vi "Timing Facade.vi"(0 "Data In":T4, 2 "Display State In":T2, 3 "Container State":T3) -> (6 "Data Out":T4, 7 "Display State Out":T2, 8 "Action":T1)   [LabVIEW 2012, in "Time Slider.xctl"]
uses:
  Time Slider.xctl
  Timing Data.ctl
  <vilib>/_xctls/Container State.ctl
  Timing State.ctl
  <vilib>/_xctls/Action.ctl
  <vilib>/_xctls/XControlSupport.lvlib
panel:
  in  "Off-Time":bool
  in  "On-Time":bool
  in  "SEQ 1":cluster{dbl, dbl, dbl}(slide) scale=0.0..20.0 scale format="%#.2f"
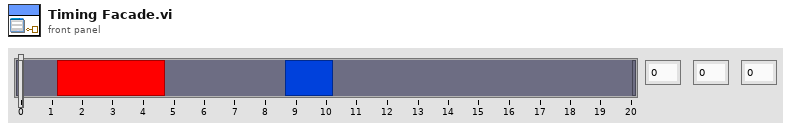
[diagram p1: front panel]
types:
  T1 = typedef "XControlSupport.lvlib/Action.ctl" = cluster{"Data Changed?":bool, "State Changed?":bool, "Action Name":string}
  T2 = typedef "Time Slider.xctl/Timing State.ctl" = cluster{"Range Max":dbl, "Range Min":dbl}
  T3 = typedef "XControlSupport.lvlib/Container State.ctl" = cluster{"Indicator?":bool, "Run Mode?":bool, " Refnum":refnum<vi>}
  T4 = typedef "Time Slider.xctl/Timing Data.ctl" = cluster{"Data":dbl, "Data 2":dbl, "Data 3":dbl}
  T5 = cluster{"Old Slider Values":dbl[], "Mouse Down Left":i32, "Old Controls Left":i32[], "Drag?":bool}
  T6 = enum8{"Enabled", "Disabled", "Disabled and Grayed Out"}
  T7 = typedef "LVPoint32TypeDef.ctl" = cluster{"Horizontal":i32, "Vertical":i32}
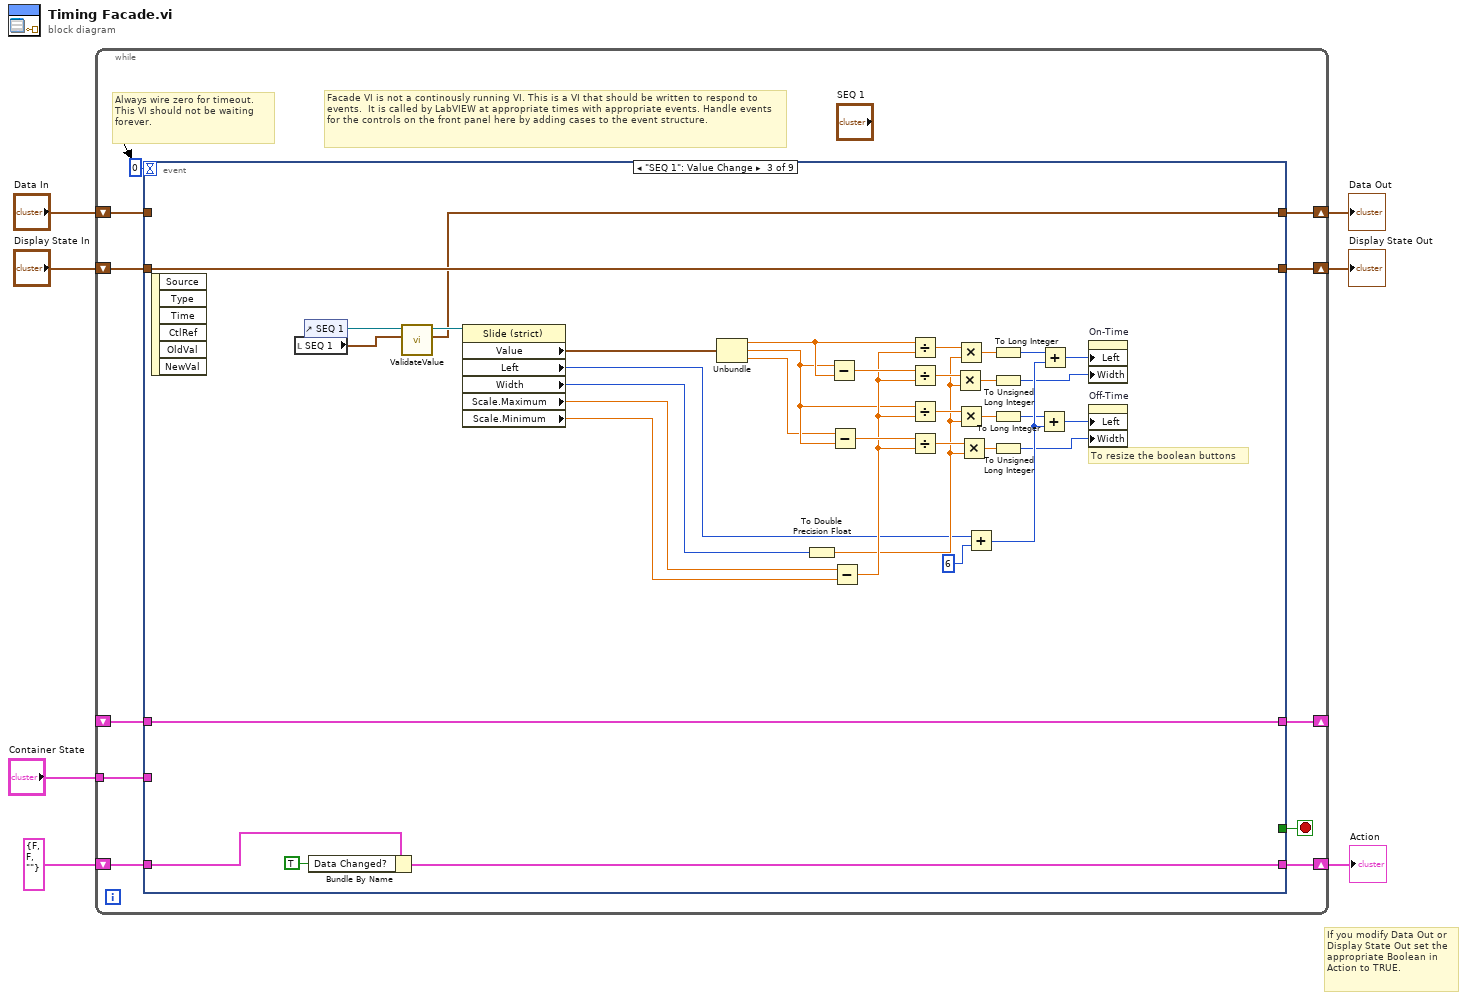
[diagram p0: block diagram]
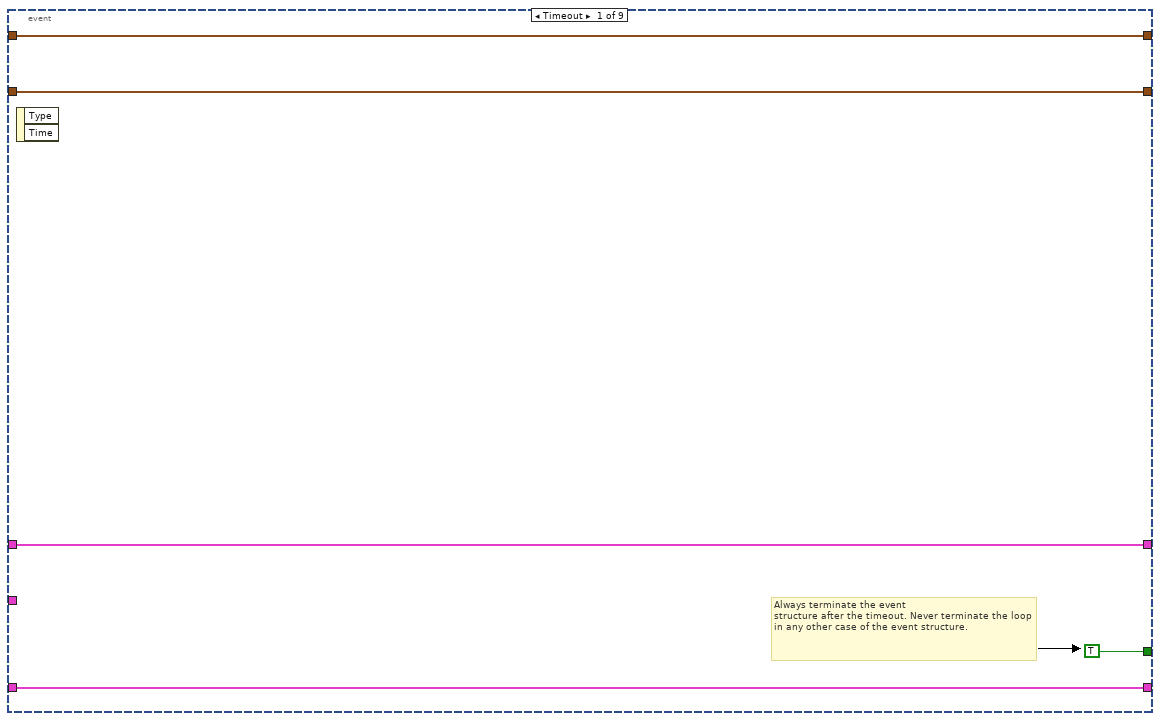
[diagram p2: hidden frame]
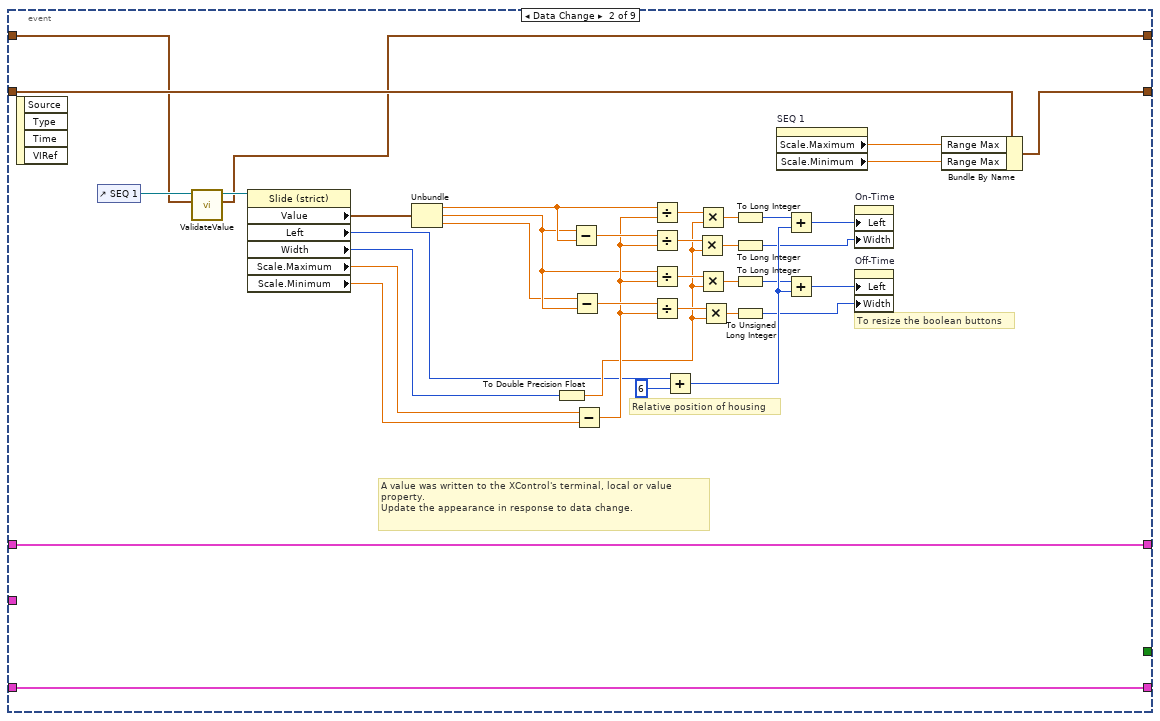
[diagram p3: hidden frame]
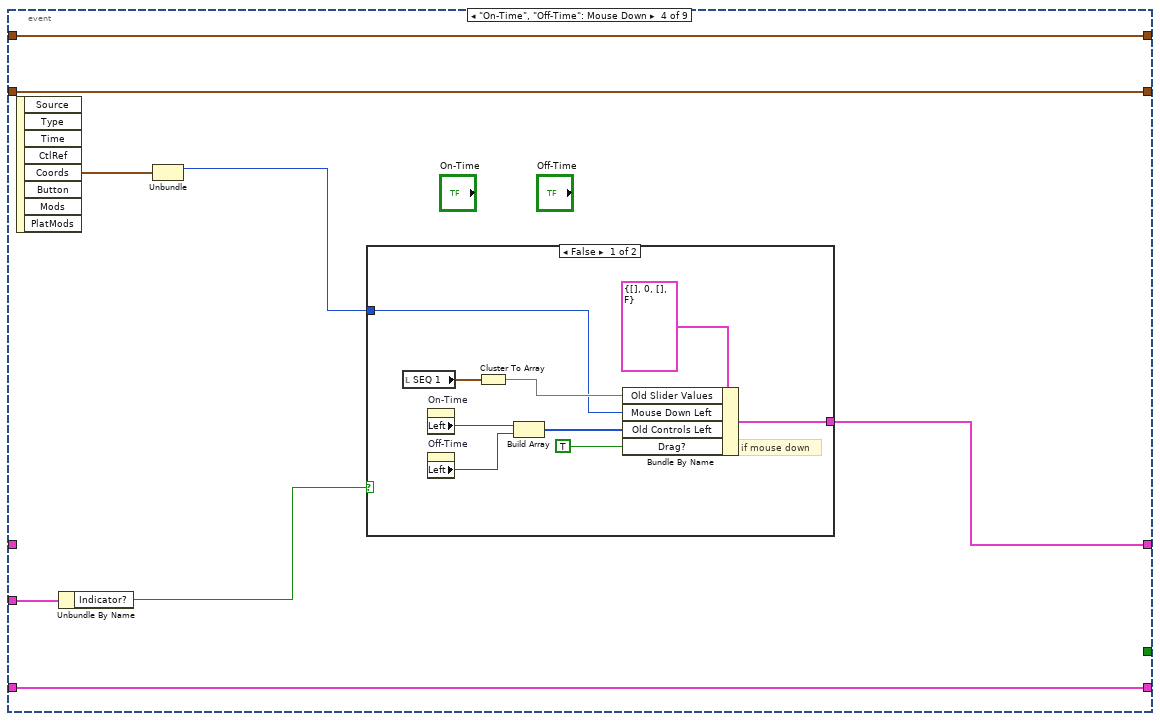
[diagram p4: hidden frame]
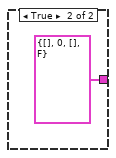
[diagram p5: hidden frame]
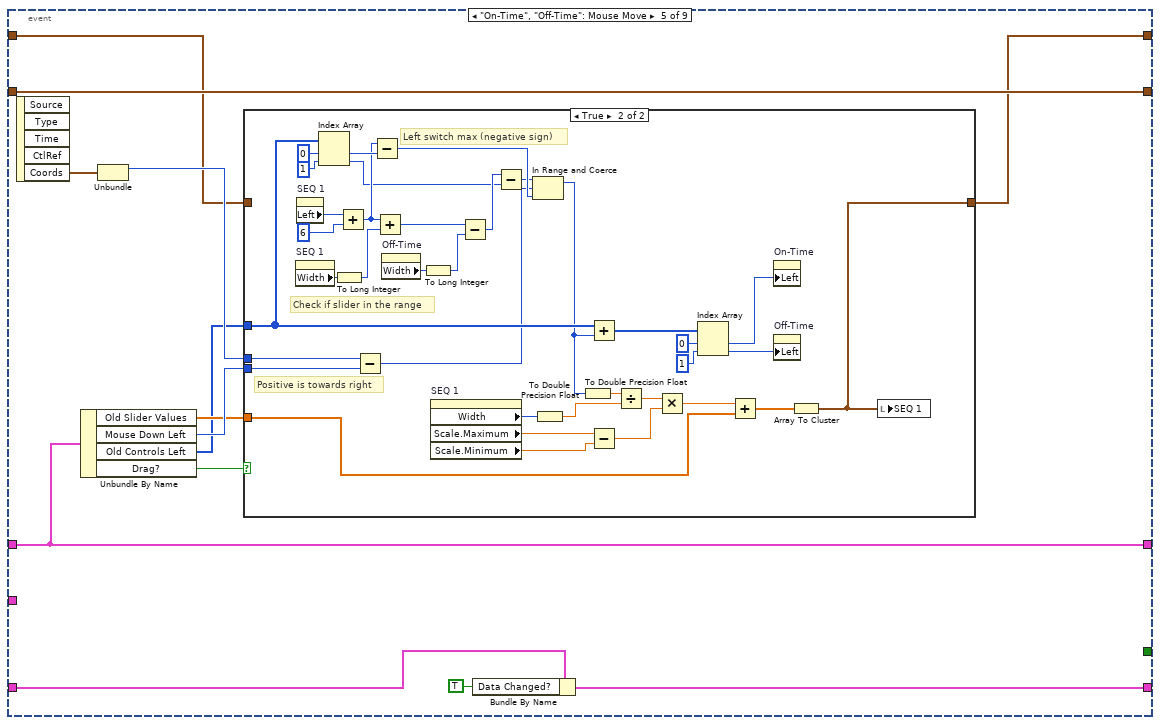
[diagram p6: hidden frame]
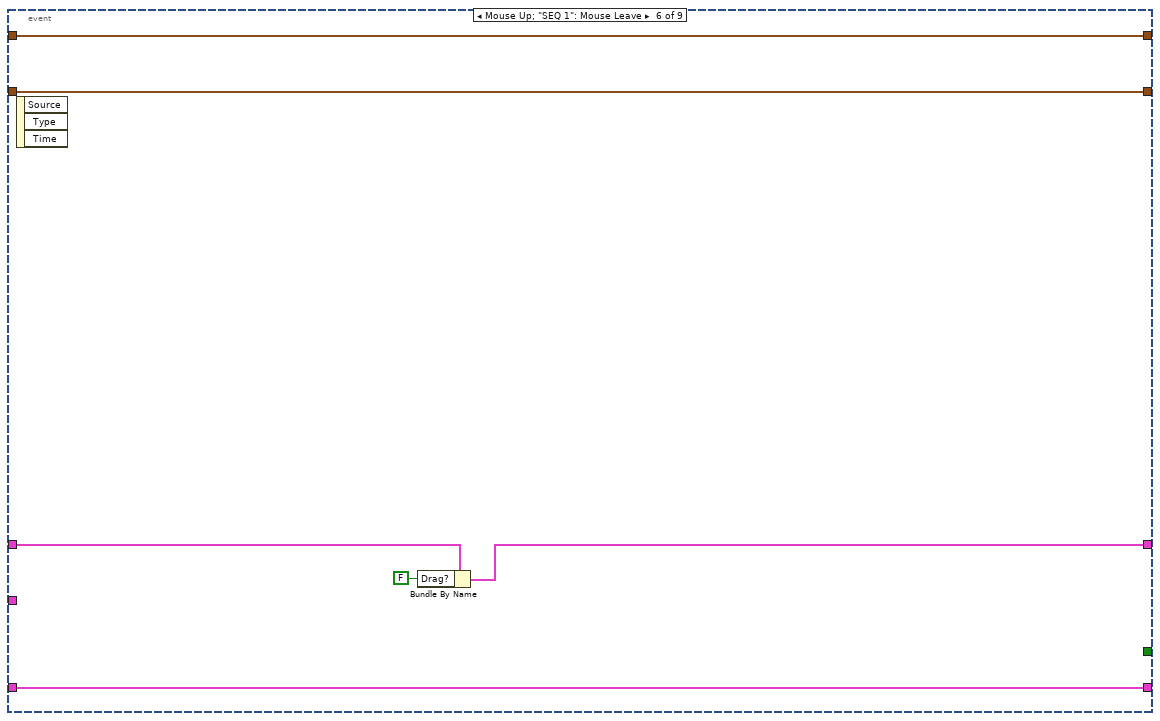
[diagram p8: hidden frame]
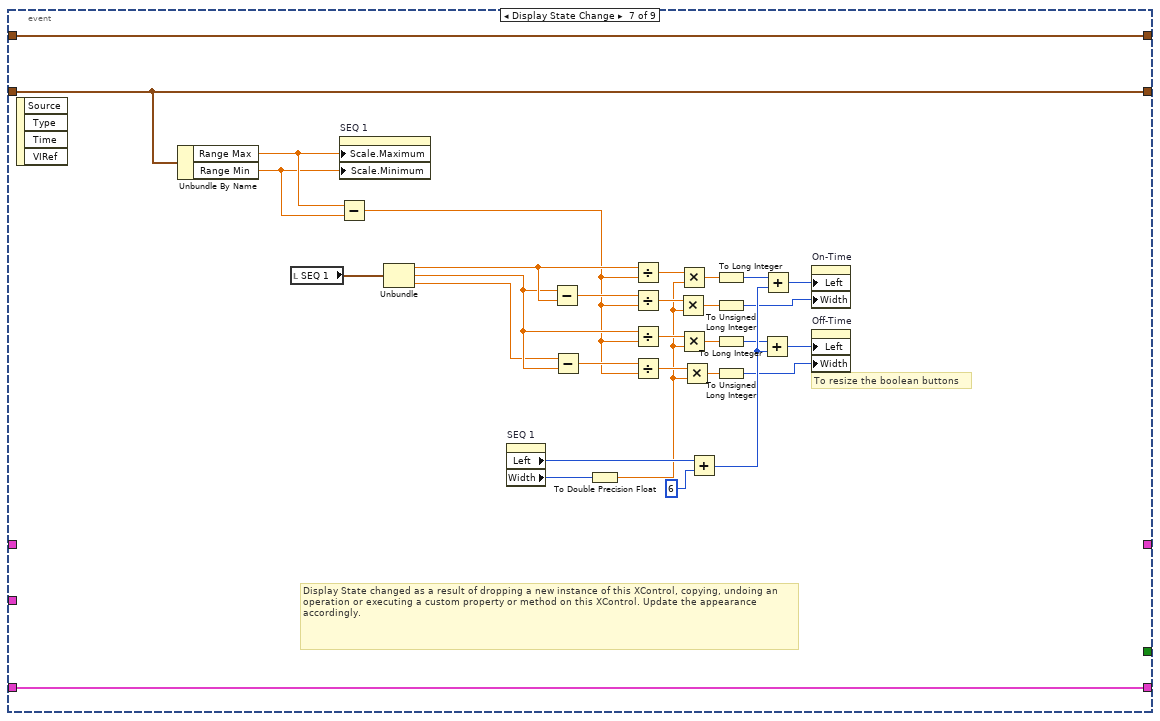
[diagram p9: hidden frame]
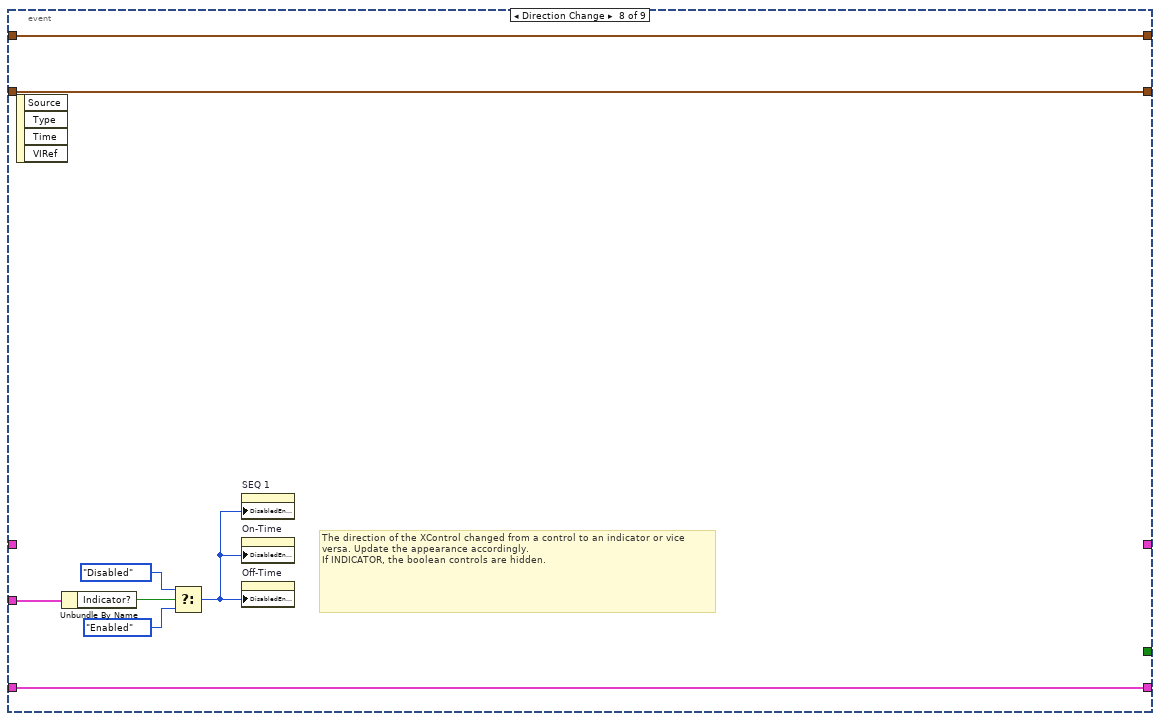
[diagram p10: hidden frame]
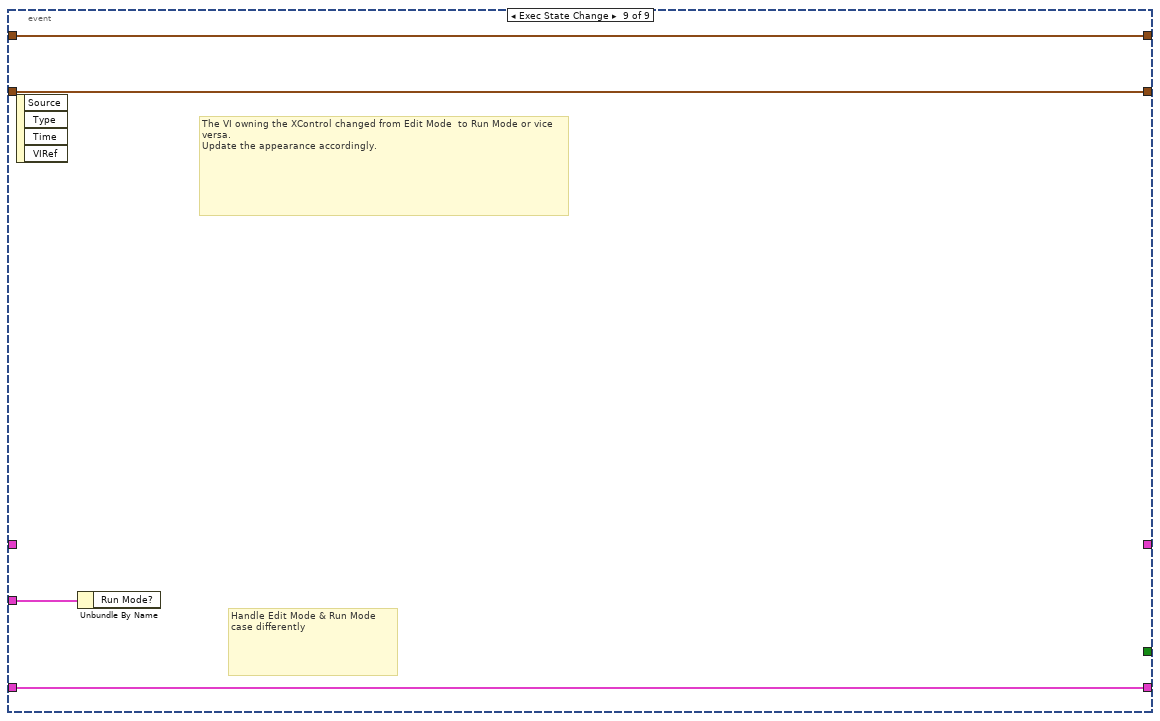
[diagram p11: hidden frame]
diagram:
  # "If you modify Data Out or Display State Out set the appropriate Boolean in Action to TRUE."
  n1 = while {
    shift-right: [w17] -> w4
    shift-left: "Display State In" -> [w18]
    tunnel: "Container State" -> [w14]
    shift-right: [w12] -> w7
    shift-left: "Data In" -> [w13]
    shift-right: [w10] -> w2
    shift-left: T1 {"Data Changed?"=FALSE, "State Changed?"=FALSE, "Action Name"=""} ("Action") -> [w11]
    shift-right: [w9] -> _
    shift-left: _ -> [w8]
    stop <- w16 stop-if-true
    # "Facade VI is not a continously running VI. This is a VI that should be written to respond to events.  It is called by LabVIEW at appropriate times with appropriate events. Handle events for the controls on the front panel here by adding cases to the event structure."
    # "Always wire zero for timeout. This VI should not be waiting forever."
    n2 = event shown="[2] \"SEQ 1\": Value Change" {
      selector: _ -> [_ _ _ _ _ _ _ _ _]
      dyn-events: _ -> [_ _ _ _ _ _ _ _ _]
      timeout: 0 -> [_ _ _ _ _ _ _ _ _]
      tunnel: w18 -> [w19 w37 w98 w106 w129 w172 w201 w210 w214]
      tunnel: [w19 w36 w98 w106 w129 w172 w201 w210 w214] -> w17
      tunnel: [TRUE _ _ _ _ _ _ _ _] -> w16
      tunnel: w14 -> [_ _ _ w103 _ _ _ w211 w215]
      tunnel: w13 -> [w21 w33 _ w104 w124 w171 w203 w209 w213]
      tunnel: [w21 w25 w63 w104 w123 w171 w203 w209 w213] -> w12
      tunnel: [w22 w61 w82 w99 w117 w167 w202 w208 w212] -> w10
      tunnel: w11 -> [w22 w61 w83 w99 w118 w167 w202 w208 w212]
      tunnel: [w20 w46 w79 w105 w121 w168 _ _ _] -> w9
      tunnel: w8 -> [w20 w46 w79 _ w121 w170 _ _ _]
      event Timeout {
        # "Always terminate the event\nstructure after the timeout. Never terminate the loop in any other case of the event structure."
        n3 = event-data() -> ()  [unwired: 1 in, 2 out]
      }
      event Data Change {
        # "Relative position of housing"
        # "To resize the boolean buttons"
        # "A value was written to the XControl's terminal, local or value property.\nUpdate the appearance in response to data change."
        n4 = event-data() -> ()  [unwired: 1 in, 4 out]
        n5 = control-ref of="SEQ 1"() -> (w34:refnum<vi>)
        n6 = call "ValidateValue.vi"("SEQ 1"=w33, "Slide Refnum in"=w34) -> ("SEQ out"=w25:cluster{dbl, dbl, dbl}, "Slide Refnum out"=w35:refnum<vi>)  [unwired: 8 in]
        n7 = property class="Slide (strict)"(reference=w35) -> ("Value"=w24:cluster{dbl, dbl, dbl}, "Left"=w29:i32, "Width"=w28:u32, "Scale.Maximum"=w27:dbl, "Scale.Minimum"=w26:dbl)  [unwired: 1 in, 2 out]
        n8 = Unbundle(w24) -> (w32:dbl, w31:dbl, w30:dbl)
        n9 = To Double Precision Float(number=w28) -> (double precision float=w45:dbl)
        n10 = Subtract(x=w31, y=w32) -> (x-y=w60:dbl)
        n11 = Subtract(x=w30, y=w31) -> (x-y=w57:dbl)
        n12 = Subtract(x=w27, y=w26) -> (x-y=w48:dbl)
        n13 = Divide(x=w32, y=w48) -> (x/y=w54:dbl)
        n14 = Divide(x=w60, y=w48) -> (x/y=w59:dbl)
        n15 = Divide(x=w31, y=w48) -> (x/y=w51:dbl)
        n16 = Divide(x=w57, y=w48) -> (x/y=w56:dbl)
        n17 = Add(x=w29, y=6) -> (x+y=w47:i32)
        n18 = Multiply(x=w59, y=w45) -> (x*y=w58:dbl)
        n19 = Multiply(x=w54, y=w45) -> (x*y=w53:dbl)
        n20 = Multiply(x=w51, y=w45) -> (x*y=w50:dbl)
        n21 = Multiply(x=w56, y=w45) -> (x*y=w55:dbl)
        n22 = To Long Integer(number=w53) -> (32bit integer=w44:i32)
        n23 = To Long Integer(number=w58) -> (32bit integer=w40:i32)
        n24 = To Long Integer(number=w50) -> (32bit integer=w42:i32)
        n25 = To Unsigned Long Integer(number=w55) -> (unsigned 32bit integer=w41:u32)
        n26 = property on="SEQ 1" class="Slide (strict)"() -> ("Scale.Maximum"=w39:dbl, "Scale.Minimum"=w38:dbl)  [unwired: 2 in, 2 out]
        n27 = Add(x=w44, y=w47) -> (x+y=w52:i32)
        n28 = Add(x=w42, y=w47) -> (x+y=w49:i32)
        n29 = property on="On-Time" class="Bool (strict)"("Left"=w52, "Width"=w40) -> ()  [unwired: 2 in, 2 out]
        n30 = property on="Off-Time" class="Bool (strict)"("Left"=w49, "Width"=w41) -> ()  [unwired: 2 in, 2 out]
        n31 = Bundle By Name(cluster=w37, "Range Max"=w39, "Range Max"=w38) -> (w36:T2)
      }
      event "SEQ 1": Value Change {
        # "To resize the boolean buttons"
        n32 = event-data() -> ()  [unwired: 1 in, 6 out]
        n33 = local read "SEQ 1"() -> (w73:cluster{dbl, dbl, dbl})
        n34 = control-ref of="SEQ 1"() -> (w72:refnum<vi>)
        n35 = Bundle By Name(cluster=w83, "Data Changed?"=TRUE) -> (w82:T1)
        n36 = call "ValidateValue.vi"("SEQ 1"=w73, "Slide Refnum in"=w72) -> ("SEQ out"=w63:cluster{dbl, dbl, dbl}, "Slide Refnum out"=w68:refnum<vi>)  [unwired: 8 in]
        n37 = property class="Slide (strict)"(reference=w68) -> ("Value"=w62:cluster{dbl, dbl, dbl}, "Left"=w67:i32, "Width"=w66:u32, "Scale.Maximum"=w65:dbl, "Scale.Minimum"=w64:dbl)  [unwired: 1 in, 2 out]
        n38 = Unbundle(w62) -> (w71:dbl, w70:dbl, w69:dbl)
        n39 = To Double Precision Float(number=w66) -> (double precision float=w78:dbl)
        n40 = Subtract(x=w70, y=w71) -> (x-y=w97:dbl)
        n41 = Subtract(x=w69, y=w70) -> (x-y=w94:dbl)
        n42 = Subtract(x=w65, y=w64) -> (x-y=w85:dbl)
        n43 = Divide(x=w71, y=w85) -> (x/y=w91:dbl)
        n44 = Divide(x=w97, y=w85) -> (x/y=w96:dbl)
        n45 = Divide(x=w70, y=w85) -> (x/y=w88:dbl)
        n46 = Divide(x=w94, y=w85) -> (x/y=w93:dbl)
        n47 = Multiply(x=w96, y=w78) -> (x*y=w95:dbl)
        n48 = Multiply(x=w91, y=w78) -> (x*y=w90:dbl)
        n49 = Multiply(x=w88, y=w78) -> (x*y=w87:dbl)
        n50 = Multiply(x=w93, y=w78) -> (x*y=w92:dbl)
        n51 = Add(x=w67, y=6) -> (x+y=w81:i32)
        n52 = To Long Integer(number=w90) -> (32bit integer=w77:i32)
        n53 = To Unsigned Long Integer(number=w95) -> (unsigned 32bit integer=w75:u32)
        n54 = To Long Integer(number=w87) -> (32bit integer=w76:i32)
        n55 = To Unsigned Long Integer(number=w92) -> (unsigned 32bit integer=w74:u32)
        n56 = Add(x=w76, y=w81) -> (x+y=w86:i32)
        n57 = Add(x=w77, y=w81) -> (x+y=w89:i32)
        n58 = property on="On-Time" class="Bool (strict)"("Left"=w89, "Width"=w75) -> ()  [unwired: 2 in, 2 out]
        n59 = property on="Off-Time" class="Bool (strict)"("Left"=w86, "Width"=w74) -> ()  [unwired: 2 in, 2 out]
      }
      event "On-Time", "Off-Time": Mouse Down {
        n60 = event-data() -> ("Coords"=w101:T7)  [unwired: 1 in, 7 out]
        n61 = Unbundle By Name(w103) -> ("Indicator?"=w102:bool)
        n62 = Unbundle(w101) -> ("Horizontal"=w100:i32)  [unwired: 1 out]
        n63 = case shown="False" w102 {
          tunnel: [w114 T5 {"Old Slider Values"=[], "Mouse Down Left"=0, "Old Controls Left"=[], "Drag?"=FALSE}] -> w105
          tunnel: w100 -> [w107 _]
          frame False {
            # "if mouse down"
            n64 = local read "SEQ 1"() -> (w108:cluster{dbl, dbl, dbl})
            n65 = property on="On-Time" class="Bool (strict)"() -> ("Left"=w112:i32)  [unwired: 2 in, 2 out]
            n66 = property on="Off-Time" class="Bool (strict)"() -> ("Left"=w111:i32)  [unwired: 2 in, 2 out]
            n67 = Cluster To Array(cluster=w108) -> (array=w109:dbl[])
            n68 = Build Array(w112, w111) -> (w110:i32[])
            n69 = Bundle By Name(cluster=T5 {"Old Slider Values"=[], "Mouse Down Left"=0, "Old Controls Left"=[], "Drag?"=FALSE}, "Old Slider Values"=w109, "Mouse Down Left"=w107, "Old Controls Left"=w110, "Drag?"=TRUE) -> (w114:T5)
          }
          frame True {
          }
        }
      }
      event "On-Time", "Off-Time": Mouse Move {
        n70 = event-data() -> ("Coords"=w128:T7)  [unwired: 1 in, 4 out]
        n71 = Unbundle By Name(w121) -> ("Old Slider Values"=w122:dbl[], "Mouse Down Left"=w125:i32, "Old Controls Left"=w120:i32[], "Drag?"=w126:bool)
        n72 = Unbundle(w128) -> ("Horizontal"=w127:i32)  [unwired: 1 out]
        n73 = case shown="True" w126 {
          tunnel: w127 -> [_ w166]
          tunnel: w125 -> [_ w165]
          tunnel: w120 -> [_ w148]
          tunnel: w124 -> [w130 _]
          tunnel: [w130 w153] -> w123
          tunnel: w122 -> [_ w152]
          frame False {
          }
          frame True {
            # "Positive is towards right"
            # "Left switch max (negative sign)"
            # "Check if slider in the range"
            n74 = property on="SEQ 1" class="Slide (strict)"() -> ("Width"=w141:u32)  [unwired: 2 in, 2 out]
            n75 = property on="SEQ 1" class="Slide (strict)"() -> ("Left"=w151:i32)  [unwired: 2 in, 2 out]
            n76 = Index Array(array=w148, index #1=0 ("index"), index #2=1 ("index")) -> (element #1=w143:i32, element #2=w137:i32)
            n77 = To Long Integer(number=w141) -> (32bit integer=w134:i32)
            n78 = Add(x=w151, y=6) -> (x+y=w142:i32)
            n79 = Subtract(x=w166, y=w165) -> (x-y=w144:i32)
            n80 = Subtract(x=w142, y=w143) -> (x-y=w145:i32)
            n81 = Add(x=w142, y=w134) -> (x+y=w139:i32)
            n82 = property on="Off-Time" class="Bool (strict)"() -> ("Width"=w140:u32)  [unwired: 2 in, 2 out]
            n83 = To Long Integer(number=w140) -> (32bit integer=w133:i32)
            n84 = property on="SEQ 1" class="Slide (strict)"() -> ("Width"=w160:u32, "Scale.Maximum"=w156:dbl, "Scale.Minimum"=w155:dbl)  [unwired: 2 in, 2 out]
            n85 = Subtract(x=w139, y=w133) -> (x-y=w138:i32)
            n86 = Subtract(x=w138, y=w137) -> (x-y=w136:i32)
            n87 = In Range and Coerce(upper limit=w136, x=w144, lower limit=w145) -> (coerced(x)=w135:i32)  [unwired: 1 out]
            n88 = To Double Precision Float(number=w160) -> (double precision float=w132:dbl)
            n89 = To Double Precision Float(number=w135) -> (double precision float=w131:dbl)
            n90 = Add(x=w148, y=w135) -> (x+y=w164:i32[])
            n91 = Subtract(x=w156, y=w155) -> (x-y=w154:dbl)
            n92 = Divide(x=w131, y=w132) -> (x/y=w159:dbl)
            n93 = Multiply(x=w159, y=w154) -> (x*y=w158:dbl)
            n94 = Index Array(array=w164, index #1=0 ("index"), index #2=1 ("index")) -> (element #1=w149:i32, element #2=w161:i32)
            n95 = Add(x=w158, y=w152) -> (x+y=w157:dbl[])
            n96 = property on="On-Time" class="Bool (strict)"("Left"=w149) -> ()  [unwired: 2 in, 2 out]
            n97 = property on="Off-Time" class="Bool (strict)"("Left"=w161) -> ()  [unwired: 2 in, 2 out]
            n98 = Array To Cluster(array=w157) -> (cluster=w153:cluster{"[0]":dbl, "[1]":dbl, "[2]":dbl})
            n99 = local write "SEQ 1"(w153) -> ()
          }
        }
        n100 = Bundle By Name(cluster=w118, "Data Changed?"=TRUE) -> (w117:T1)
      }
      event Mouse Up; "SEQ 1": Mouse Leave {
        n101 = event-data() -> ()  [unwired: 1 in, 3 out]
        n102 = Bundle By Name(cluster=w170, "Drag?"=FALSE) -> (w168:T5)
      }
      event Display State Change {
        # "To resize the boolean buttons"
        # "Display State changed as a result of dropping a new instance of this XControl, copying, undoing an operation or executing a custom property or method on this XControl. Update the appearance accordingly."
        n103 = event-data() -> ()  [unwired: 1 in, 4 out]
        n104 = Unbundle By Name(w201) -> ("Range Max"=w175:dbl, "Range Min"=w174:dbl)
        n105 = local read "SEQ 1"() -> (w179:cluster{dbl, dbl, dbl})
        n106 = Subtract(x=w175, y=w174) -> (x-y=w173:dbl)
        n107 = property on="SEQ 1" class="Slide (strict)"("Scale.Maximum"=w175, "Scale.Minimum"=w174) -> ()  [unwired: 2 in, 2 out]
        n108 = Unbundle(w179) -> (w178:dbl, w177:dbl, w176:dbl)
        n109 = property on="SEQ 1" class="Slide (strict)"() -> ("Left"=w187:i32, "Width"=w188:u32)  [unwired: 2 in, 2 out]
        n110 = Subtract(x=w177, y=w178) -> (x-y=w200:dbl)
        n111 = Subtract(x=w176, y=w177) -> (x-y=w197:dbl)
        n112 = To Double Precision Float(number=w188) -> (double precision float=w184:dbl)
        n113 = Divide(x=w178, y=w173) -> (x/y=w194:dbl)
        n114 = Divide(x=w200, y=w173) -> (x/y=w199:dbl)
        n115 = Divide(x=w177, y=w173) -> (x/y=w191:dbl)
        n116 = Divide(x=w197, y=w173) -> (x/y=w196:dbl)
        n117 = Multiply(x=w199, y=w184) -> (x*y=w198:dbl)
        n118 = Multiply(x=w194, y=w184) -> (x*y=w193:dbl)
        n119 = Multiply(x=w191, y=w184) -> (x*y=w190:dbl)
        n120 = Multiply(x=w196, y=w184) -> (x*y=w195:dbl)
        n121 = Add(x=w187, y=6) -> (x+y=w186:i32)
        n122 = To Long Integer(number=w193) -> (32bit integer=w183:i32)
        n123 = To Unsigned Long Integer(number=w198) -> (unsigned 32bit integer=w181:u32)
        n124 = To Long Integer(number=w190) -> (32bit integer=w182:i32)
        n125 = To Unsigned Long Integer(number=w195) -> (unsigned 32bit integer=w180:u32)
        n126 = Add(x=w182, y=w186) -> (x+y=w189:i32)
        n127 = Add(x=w183, y=w186) -> (x+y=w192:i32)
        n128 = property on="On-Time" class="Bool (strict)"("Left"=w192, "Width"=w181) -> ()  [unwired: 2 in, 2 out]
        n129 = property on="Off-Time" class="Bool (strict)"("Left"=w189, "Width"=w180) -> ()  [unwired: 2 in, 2 out]
      }
      event Direction Change {
        # "The direction of the XControl changed from a control to an indicator or vice versa. Update the appearance accordingly.\nIf INDICATOR, the boolean controls are hidden."
        n130 = event-data() -> ()  [unwired: 1 in, 4 out]
        n131 = Unbundle By Name(w211) -> ("Indicator?"=w207:bool)
        n132 = Select(t=T6."Disabled" ("Disabled"), s=w207, f=T6."Enabled" ("Disabled")) -> (s? t:f=w204:T6)
        n133 = property on="SEQ 1" class="Slide (strict)"("DisabledEnum"=w204) -> ()  [unwired: 2 in, 2 out]
        n134 = property on="On-Time" class="Bool (strict)"("DisabledEnum"=w204) -> ()  [unwired: 2 in, 2 out]
        n135 = property on="Off-Time" class="Bool (strict)"("DisabledEnum"=w204) -> ()  [unwired: 2 in, 2 out]
      }
      event Exec State Change {
        # "The VI owning the XControl changed from Edit Mode  to Run Mode or vice versa.\nUpdate the appearance accordingly."
        # "Handle Edit Mode & Run Mode\ncase differently"
        n136 = event-data() -> ()  [unwired: 1 in, 4 out]
        n137 = Unbundle By Name(w215) -> ()  [unwired: 1 out]
      }
    }
  }
  "Display State Out" <- w4
  "Data Out" <- w7
  "Action" <- w2
